vi "get_status_from_zc.vi"(10 "zc_luodi_num":string) -> (0 "error":errorcluster caption="error out 4", 2 "status":string)   [LabVIEW 2017, in "Lib_code.lvlib"]
uses:
  Lib_code.lvlib
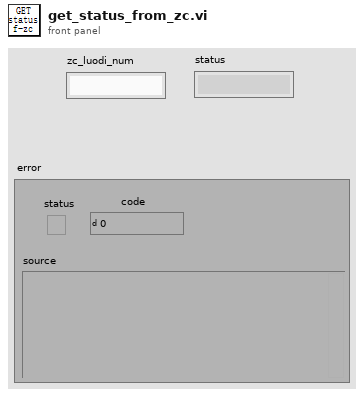
[diagram p1: front panel]
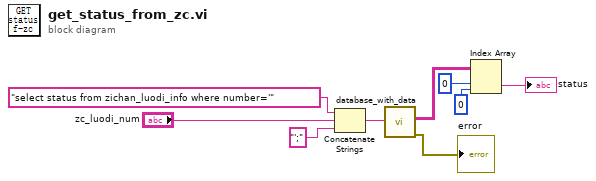
[diagram p0: block diagram]
diagram:
  n1 = Concatenate Strings("select status from zichan_luodi_info where number='" ("字符串"), "zc_luodi_num", "';" ("字符串")) -> (w4:string)
  n2 = call "database_with_data.vi"("input"=w4) -> ("error"=→"error":errorcluster, "Data"=w2:string[][])  [unwired: 9 in]
  n3 = Index Array(array=w2, index (row)=0 ("索引 (行)"), index (col)=0 ("禁用的索引 (列)")) -> (element=→"status":string)
